vi "Step Response(Loop).vi"() -> ()   [LabVIEW 2019]
uses:
  ADC_CTRL.ctl
  <userlib>/Common_VIs/Instrument/Supply/Channel Control.ctl
panel:
  out "Array":T2(array[cluster])
  in  "Supply_VDDA":refnum<visa-resource-name>="GPIB0::2::INSTR"
  out "error out":errorcluster
  in  "file path (dialog if empty)":path
  in  "Supply_Input":refnum<visa-resource-name>="GPIB0::2::INSTR"
  in  "Supply_Reference":refnum<visa-resource-name>="GPIB0::2::INSTR"
  in  "error in":errorcluster
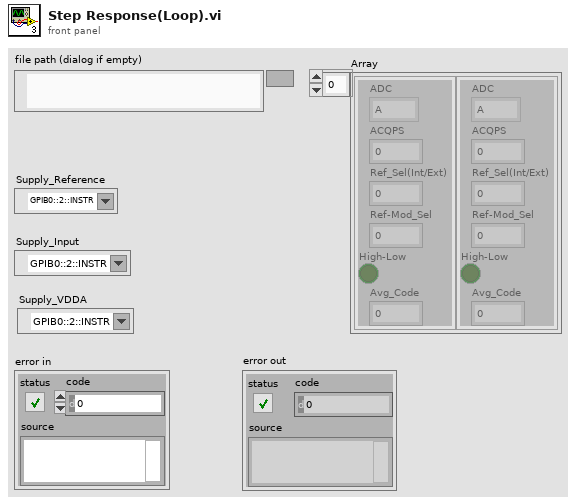
[diagram p1: front panel]
types:
  T1 = typedef "ADC_CTRL.ctl" = enum16{"A", "B", "C"}
  T2 = cluster{"ADC":T1, "ACQPS":u16, "Ref_Sel(Int/Ext)":u16, "Ref-Mod_Sel":u16, "High-Low":bool, "Avg_Code":dbl}[]
  T3 = cluster{"Voltage":dbl, "Current Limit":dbl, "Configure ":bool}
  T4 = typedef "Channel Control.ctl" = cluster{"Output ?":bool, "Enable":bool, "Voltage Level (V)":dbl, "Current Limit (A) ":dbl}
  T5 = cluster{"ADC":T1, "ACQPS":u16, "Ref_Sel(Int/Ext)":u16, "Ref-Mod_Sel":u16, "High-Low":bool, "Avg_Code":dbl}
  T6 = cluster{"ACQPS":u16, "Ref_Sel(Int/Ext)":u16, "Break_PT":u16, "Ref-Mode_Sel":u16}
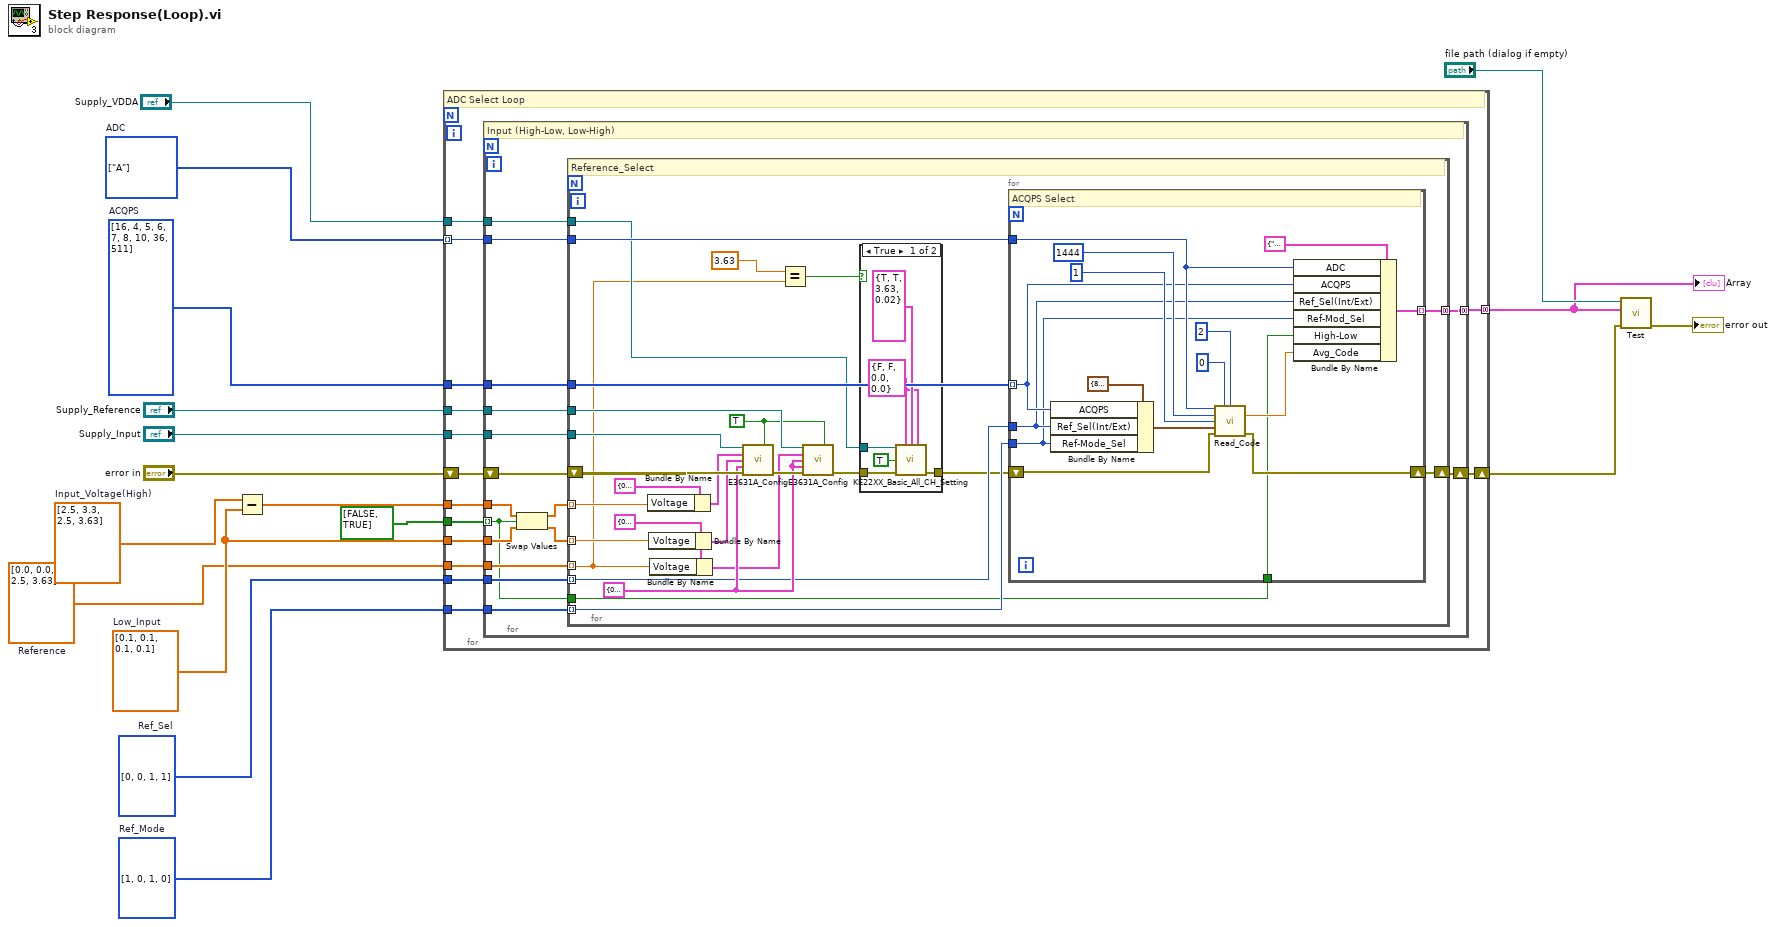
[diagram p0: block diagram]
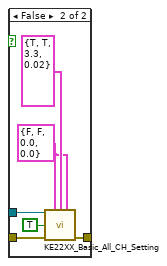
[diagram p2: hidden frame]
diagram:
  w7 = dbl[] [0.0, 0.0, 2.5, 3.63]  # Reference
  w11 = dbl[] [0.1, 0.1, 0.1, 0.1]  # Low_Input
  w9 = u16[] [1, 0, 1, 0]  # Ref_Mode
  w6 = dbl[] [2.5, 3.3, 2.5, 3.63]  # Input_Voltage(High)
  w10 = u16[] [0, 0, 1, 1]  # Ref_Sel
  w16 = u16[] [16, 4, 5, 6, 7, 8, 10, 36, 511]  # ACQPS
  w17 = T1[] [enum."A"] items=["A", "B", "C"]  # ADC
  n1 = Subtract(x=w6, y=w11) -> (x-y=w12:dbl[])
  n2 = for {
    tunnel: w17 -> [w31] mode=indexing
    tunnel: w16 -> [w30]
    tunnel: "Supply_Reference" -> [w28]
    tunnel: "Supply_Input" -> [w27]
    shift-right: [w26] -> w4
    shift-left: "error in" -> [w29]
    tunnel: w12 -> [w25]
    tunnel: w11 -> [w24]
    tunnel: w10 -> [w23]
    tunnel: w9 -> [w22]
    tunnel: bool[] [FALSE, TRUE] -> [w21]
    tunnel: w7 -> [w20]
    tunnel: [w19] -> w1 mode=concatenating
    tunnel: "Supply_VDDA" -> [w18]
    # "ADC Select Loop"
    n3 = for {
      tunnel: w31 -> [w47]
      tunnel: w30 -> [w46]
      tunnel: w28 -> [w45]
      tunnel: w27 -> [w43]
      shift-right: [w44] -> w26
      shift-left: w29 -> [w42]
      tunnel: w25 -> [w39]
      tunnel: w24 -> [w38]
      tunnel: w23 -> [w41]
      tunnel: w22 -> [w40]
      tunnel: w21 -> [w32] mode=indexing
      tunnel: w20 -> [w35]
      tunnel: [w34] -> w19 mode=concatenating
      tunnel: w18 -> [w33]
      # "Input (High-Low, Low-High)"
      n4 = Swap Values(12:w39, 13:w32, 14:w38) -> (1:w36:dbl[], 3:w37:dbl[])
      n5 = for {
        tunnel: w47 -> [w73]
        tunnel: w46 -> [w72]
        tunnel: w45 -> [w71]
        shift-right: [w70] -> w44
        shift-left: w42 -> [w67]
        tunnel: w43 -> [w69]
        tunnel: w36 -> [w66] mode=indexing
        tunnel: w37 -> [w62] mode=indexing
        tunnel: w41 -> [w59] mode=indexing
        tunnel: w40 -> [w58] mode=indexing
        tunnel: w35 -> [w51] mode=indexing
        tunnel: [w55] -> w34 mode=concatenating
        tunnel: w33 -> [w53]
        tunnel: w32 -> [w48]
        w60 = TRUE ("Enable Output")
        w61 = T3 {"Voltage"=0.0, "Current Limit"=0.05, "Configure "=FALSE} ("Channel_3")
        w56 = T3 {"Voltage"=0.0, "Current Limit"=0.01, "Configure "=TRUE} ("Channel_3")
        # "Reference_Select"
        n6 = Bundle By Name(cluster=T3 {"Voltage"=0.0, "Current Limit"=0.01, "Configure "=TRUE} ("Channel_1"), "Voltage"=w66) -> (w64:T3)
        n7 = Bundle By Name(cluster=w56, "Voltage"=w62) -> (w65:T3)
        n8 = Bundle By Name(cluster=w56, "Voltage"=w51) -> (w57:T3)
        n9 = call <userlib>:"E3631A_Config.vi"("VISA resource name"=w69, "Enable Output"=w60, "Channel_1"=w64, "Channel_2"=w65, "Channel_3"=w61, "error in (no error)"=w67) -> ("error out"=w68:errorcluster)  [unwired: 8 in, 1 out]
        n10 = Equal?(x=3.63, y=w51) -> (x = y?=w52:bool)
        n11 = call <userlib>:"E3631A_Config.vi"("VISA resource name"=w71, "Enable Output"=w60, "Channel_1"=w57, "Channel_2"=w61, "Channel_3"=w61, "error in (no error)"=w68) -> ("error out"=w54:errorcluster)  [unwired: 8 in, 1 out]
        n12 = case shown="True" w52 {
          tunnel: w54 -> [w78 w82]
          tunnel: w53 -> [w79 w83]
          tunnel: [w77 w80] -> w49
          frame True {
            w75 = T4 {"Output ?"=FALSE, "Enable"=FALSE, "Voltage Level (V)"=0.0, "Current Limit (A) "=0.0} ("Channe 1")
            n13 = call <userlib>:"KE22XX_Basic_All_CH_Setting.vi"("VISA In"=w79, "Channe 1"=w75, "Channe 2"=T4 {"Output ?"=TRUE, "Enable"=TRUE, "Voltage Level (V)"=3.63, "Current Limit (A) "=0.02}, "Channe 3"=w75, "Remote"=TRUE, "error in"=w78) -> ("error out"=w77:errorcluster)  [unwired: 9 in]
          }
          frame False {
            w84 = T4 {"Output ?"=FALSE, "Enable"=FALSE, "Voltage Level (V)"=0.0, "Current Limit (A) "=0.0} ("Channe 1")
            n14 = call <userlib>:"KE22XX_Basic_All_CH_Setting.vi"("VISA In"=w83, "Channe 1"=w84, "Channe 2"=T4 {"Output ?"=TRUE, "Enable"=TRUE, "Voltage Level (V)"=3.3, "Current Limit (A) "=0.02}, "Channe 3"=w84, "Remote"=TRUE, "error in"=w82) -> ("error out"=w80:errorcluster)  [unwired: 9 in]
          }
        }
        n15 = for {
          tunnel: w73 -> [w93]
          tunnel: w72 -> [w92] mode=indexing
          shift-right: [w95] -> w70
          shift-left: w49 -> [w94]
          tunnel: w59 -> [w91]
          tunnel: w58 -> [w90]
          tunnel: [w88] -> w55 mode=indexing
          tunnel: w48 -> [w86]
          # "ACQPS Select"
          n16 = Bundle By Name(cluster=T6 {"ACQPS"=8, "Ref_Sel(Int/Ext)"=1, "Break_PT"=0, "Ref-Mode_Sel"=0} ("ADC_Controls"), "ACQPS"=w92, "Ref_Sel(Int/Ext)"=w91, "Ref-Mode_Sel"=w90) -> (w96:T6)
          n17 = call "Read_Code.vi"("ADC"=w93, "Device_no"=u16 0, "Repeat"=2, "Port_No"=u16 1444, "Core_No"=u16 1, "ADC_Controls"=w96, "error in"=w94) -> ("AvgCode"=w87:dbl, "error out"=w95:errorcluster)  [unwired: 7 in]
          n18 = Bundle By Name(cluster=T5 {"ADC"=enum."A", "ACQPS"=0, "Ref_Sel(Int/Ext)"=0, "Ref-Mod_Sel"=0, "High-Low"=FALSE, "Avg_Code"=0.0}, "ADC"=w93, "ACQPS"=w92, "Ref_Sel(Int/Ext)"=w91, "Ref-Mod_Sel"=w90, "High-Low"=w86, "Avg_Code"=w87) -> (w88:T5)
        }
      }
    }
  }
  "Array" <- w1
  n19 = call "Test.vi"("error constant"=w4, "Array"=w1, "file path (dialog if empty)"="file path (dialog if empty)") -> ("error out"=→"error out":errorcluster)  [unwired: 8 in]
